vi "robo_preso.vi"(8 "Robot in":T1, 10 "IA State":T6={"our_robots"=[], "enemy_robots"=[], "balls"=[], "geometry"={"field_length"=0, "field_width"=0, "goal_width"=0, "goal_depth"=0, "center_circle_radius"=0, "defense_width"=0, "defense_depth"=0, "free_kick_from_defense_dist"=0, "penalty_spot_from_field_line_dist"=0, "penalty_line_from_spot_dist"=0, "half_moon_depth"=0, "half_moon_width"=0}, "IA Judge"={"stage"="", "command"="", "our_goalie_id"=0.0, "enemy_goalie_id"=0.0, "command enum"=enum."Halt", "Time"=enum."Azul"}, "Received Timestamp"=timestamp(0 s since 1904-01-01), "Events"={"Touch"=FALSE, "id touch"=0.0, "Ball out of \nVision"=FALSE, "Ball inside \nGoalie area"=FALSE, "Robot not responding"=FALSE, "Robots responding status"=[1.0, 1.0, 1.0, 1.0, 1.0, 1.0], "Enemy Ball \nPossession"=FALSE, "Id ini Possession"=0.0, "Ball Possesion"=FALSE, "Id Possesion"=0.0, "Ball at\nour goal side"=FALSE, "Ball at\ntouchline"=FALSE, "Ball at\nenemy goal side"=FALSE}}, 11 "balls":T7[](array[typedef])) -> (1 "result":bool, 3 "Robot out":T1)   [LabVIEW 2018]
uses:
  Core/AI Ball.ctl
  Core/AI Robot.ctl
  Functions Enum.ctl
  AttackerStates.ctl
  Path Planning/RRT/PathDests.ctl
  Path Planning/RRT/PathDest.ctl
  Core/AI Input.ctl
  Core/Field Size.ctl
  Core/AI Judge.ctl
  Command Enum.ctl
  Util/Events/Events.ctl
  <vilib>/Analysis/_algsub.llb/Real Vector Norm.vi
  <vilib>/Analysis/NI_AALPro.lvlib
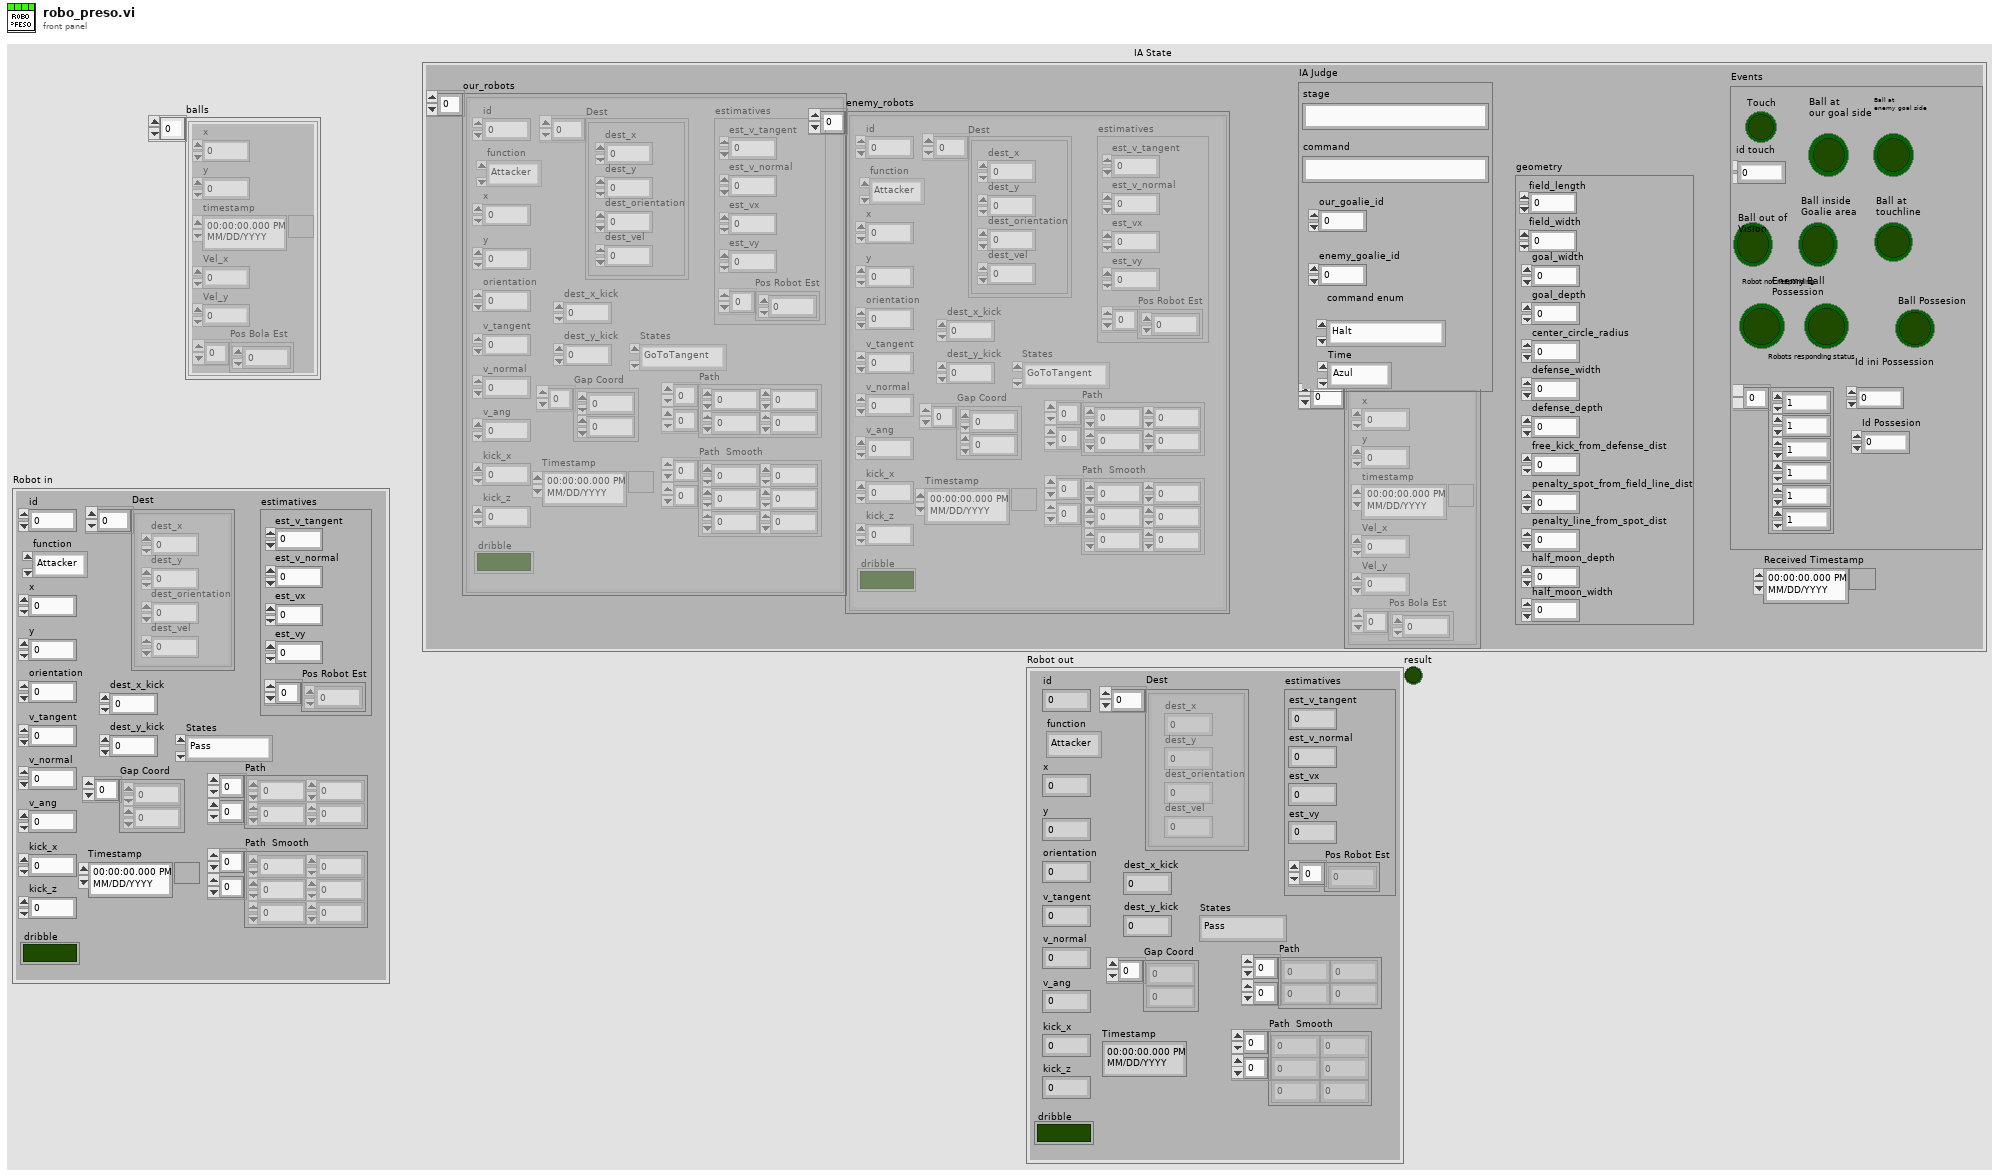
[diagram p1: front panel]
types:
  T1 = typedef "AI Robot.ctl" = cluster{"id":u32, "function":T2, "x":dbl, "y":dbl, "orientation":dbl, "v_tangent":dbl, "v_normal":dbl, "v_ang":dbl, "kick_x":dbl, "kick_z":dbl, "dribble":bool, "Timestamp":timestamp, "estimatives":cluster{"est_v_tangent":dbl, "est_v_normal":dbl, "est_vx":dbl, "est_vy":dbl, "Pos Robot Est":dbl[]}, "dest_x_kick":dbl, "dest_y_kick":dbl, "Gap Coord":dbl[], "States":T3, "Path ":dbl[][], "Path  Smooth":dbl[][], "Dest":T4}
  T2 = typedef "Functions Enum.ctl" = enum16{"Attacker", "Goalie", "Defender", "Striker", "Goto 0", "Dummy", "Kicker", "ZigZag"}
  T3 = typedef "AttackerStates.ctl" = enum16{"Pass", "GoToTangent", "BallGetting", "GoToKick", "Rotate anti-clockwise", "Rotate Clockwise", ""}
  T4 = typedef "PathDests.ctl" = T5[]
  T5 = typedef "PathDest.ctl" = cluster{"dest_x":dbl, "dest_y":dbl, "dest_orientation":dbl, "dest_vel":dbl}
  T6 = typedef "AI Input.ctl" = cluster{"our_robots":T1[], "enemy_robots":T1[], "balls":T7[], "geometry":T8, "IA Judge":T9, "Received Timestamp":timestamp, "Events":T11}
  T7 = typedef "AI Ball.ctl" = cluster{"x":dbl, "y":dbl, "timestamp":timestamp, "Vel_x":dbl, "Vel_y":dbl, "Pos Bola Est":dbl[]}
  T8 = typedef "Field Size.ctl" = cluster{"field_length":u32, "field_width":u32, "goal_width":u32, "goal_depth":u32, "center_circle_radius":u32, "defense_width":u32, "defense_depth":u32, "free_kick_from_defense_dist":u32, "penalty_spot_from_field_line_dist":u32, "penalty_line_from_spot_dist":u32, "half_moon_depth":u32, "half_moon_width":u32}
  T9 = typedef "AI Judge.ctl" = cluster{"stage":string, "command":string, "our_goalie_id":dbl, "enemy_goalie_id":dbl, "command enum":T10, "Time":enum16{"Azul", "Amarelo"}}
  T10 = typedef "Command Enum.ctl" = enum16{"Halt", "Stop", "Force Start", "PKA Normal Start", "Prepare Kickoff Ally", "PKE Normal Start", "Prepare Kickoff Enemy", "Prepare Penalty Ally", "PPA Normal Start", "Prepare Penalty Enemy", "PPE Normal Start", "Ball Placement Enemy Up", "Ball Placement Enemy Down", "Ball Placement Ally Up", "Ball Placement Ally Mid", "Ball Placement Ally Down", "Indirect Free Enemy", "Indirect Free Ally", "Timeout Enemy", "Timeout Ally", "Goal Enemy", "Goal Ally", "Normal Half Time", "Extra Time Break", "Extra Half Time", "None", "Post Game"}
  T11 = typedef "Events.ctl" = cluster{"Touch":bool, "id touch":dbl, "Ball out of \nVision":bool, "Ball inside \nGoalie area":bool, "Robot not responding":bool, "Robots responding status":dbl[], "Enemy Ball \nPossession":bool, "Id ini Possession":dbl, "Ball Possesion":bool, "Id Possesion":dbl, "Ball at\nour goal side":bool, "Ball at\ntouchline":bool, "Ball at\nenemy goal side":bool}
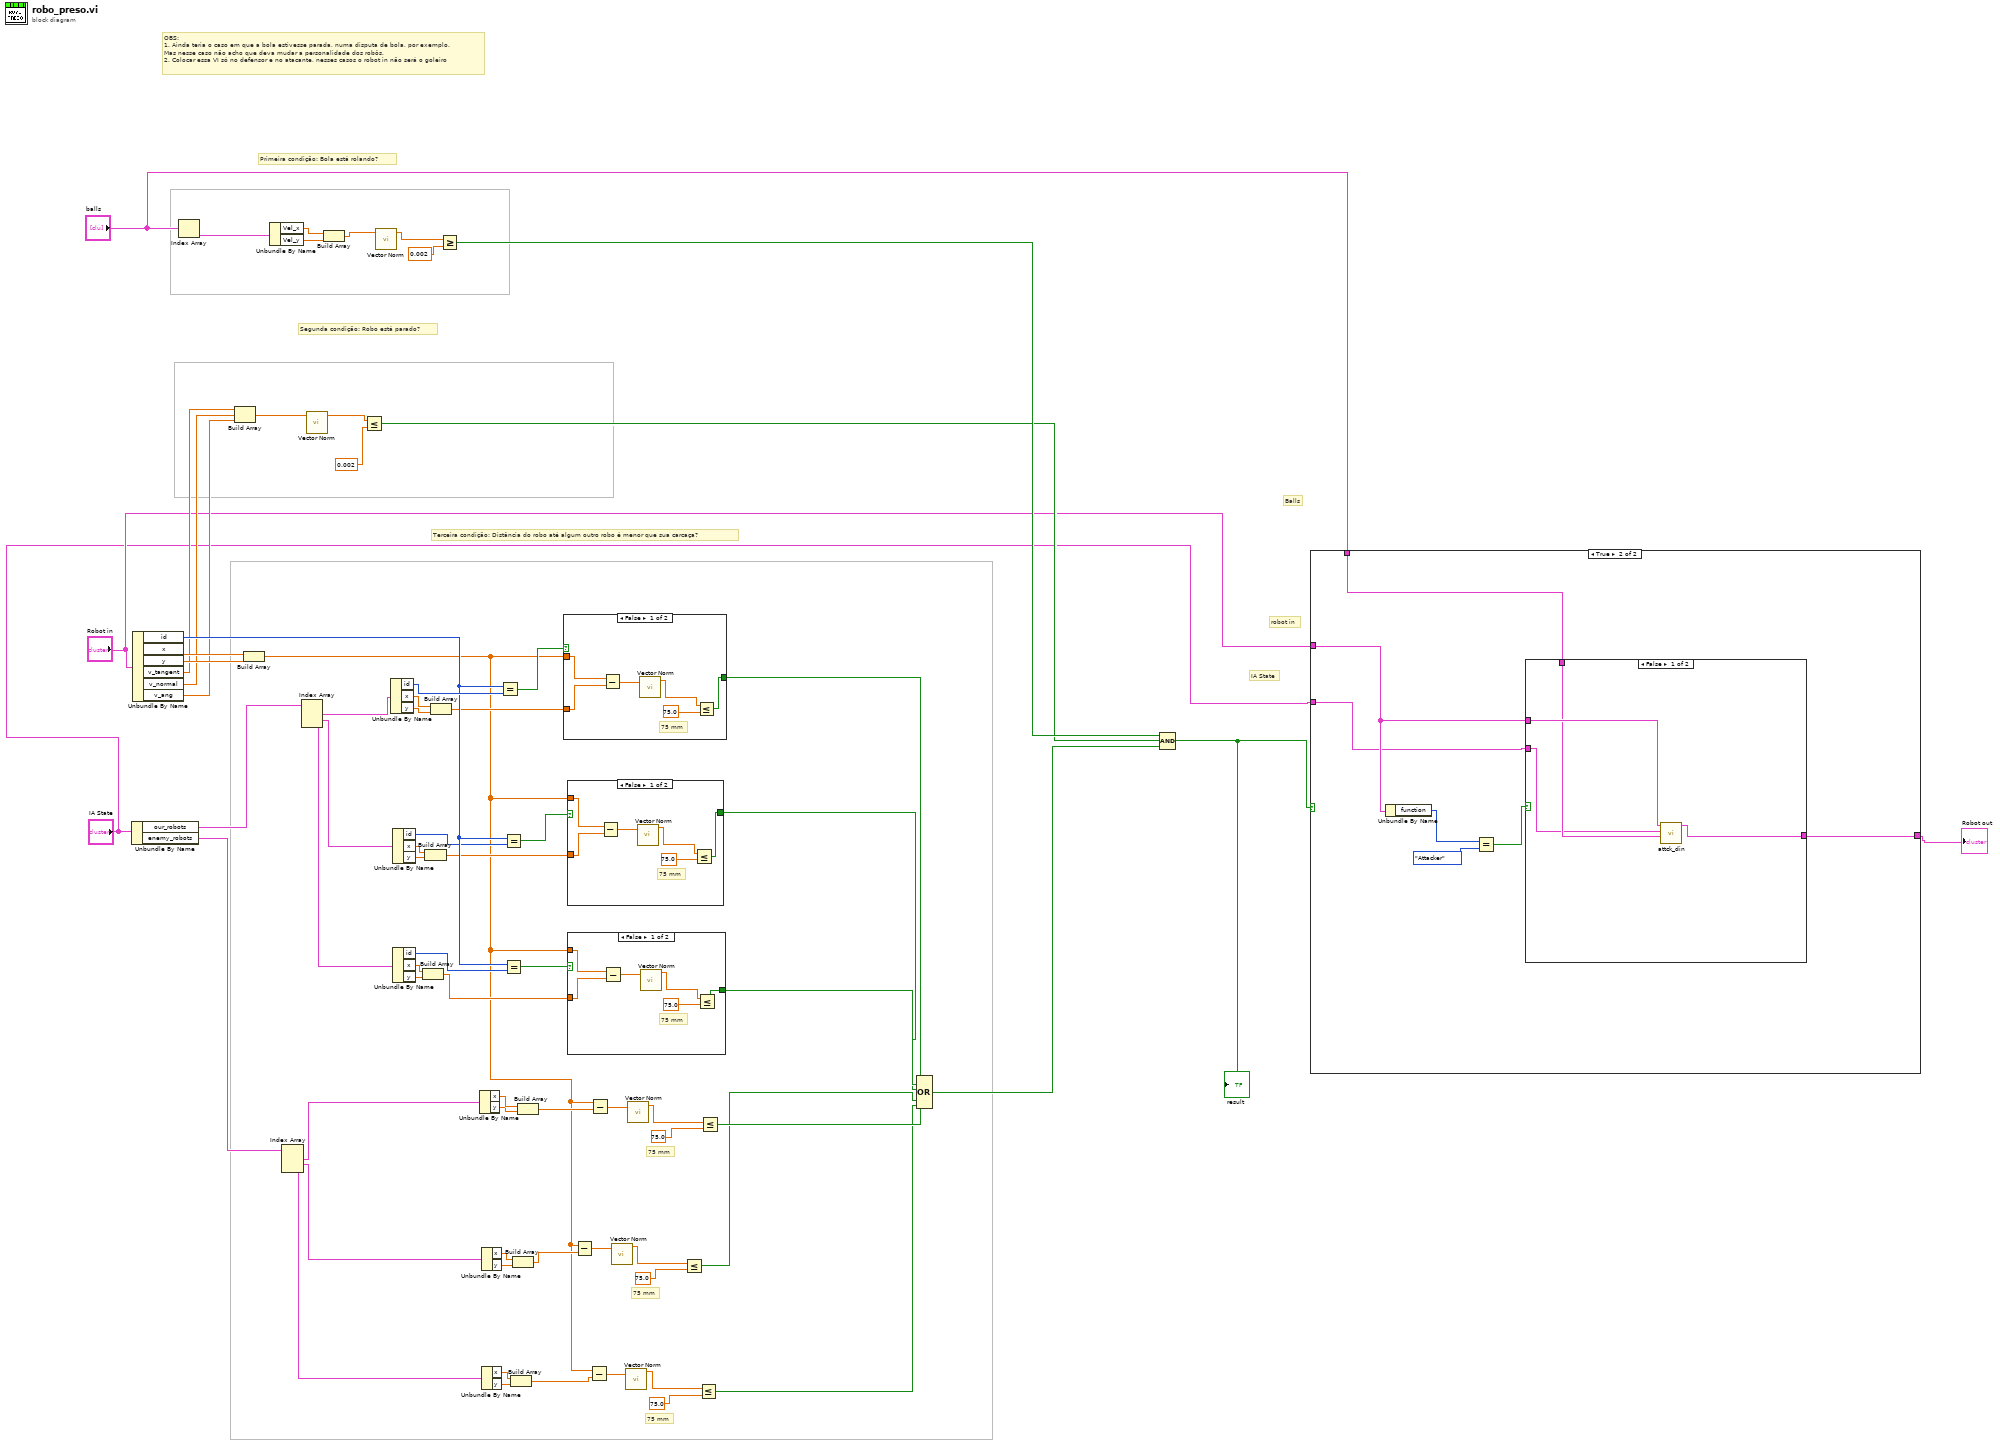
[diagram p0: block diagram]
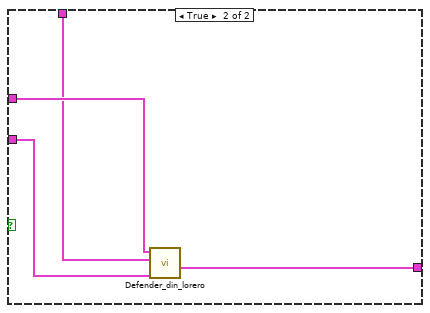
[diagram p3: hidden frame]
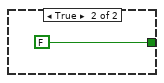
[diagram p4: hidden frame]
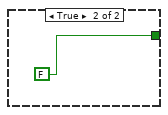
[diagram p5: hidden frame]
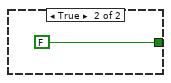
[diagram p6: hidden frame]
diagram:
  # "IA State"
  # "Balls"
  # "robot in"
  # "OBS:\n1. Ainda teria o caso em que a bola estivesse parada, numa disputa de bola, por exemplo.\nMas nesse caso não acho que deva mudar a personalidade dos robôs.\n2. Colocar essa VI só no defensor e no atacante, nesses casos o robot in não será o goleiro"
  # "Segunda condição: Robo está parado?"
  # "75 mm"
  # "75 mm"
  # "75 mm"
  # "Terceira condição: Distância do robo até algum outro robo é menor que sua carcaça?"
  # "Primeira condição: Bola está rolando?"
  n1 = Unbundle By Name("IA State") -> ("our_robots"=w5:T1[], "enemy_robots"=w33:T1[])
  n2 = Unbundle By Name("Robot in") -> ("id"=w60:u32, "x"=w54:dbl, "y"=w53:dbl, "v_tangent"=w14:dbl, "v_normal"=w13:dbl, "v_ang"=w12:dbl)
  n3 = Index Array(array="balls") -> (element=w71:T7)  [unwired: 1 in]
  n4 = Build Array(w14, w13, w12) -> (w11:dbl[])
  n5 = Build Array(w54, w53) -> (w19:dbl[])
  n6 = Unbundle By Name(w71) -> ("Vel_x"=w70:dbl, "Vel_y"=w69:dbl)
  n7 = Index Array(array=w33) -> (element #1=w34:T1, element #2=w32:T1, element #3=w31:T1)  [unwired: 3 in]
  n8 = Index Array(array=w5) -> (element #1=w62:T1, element #2=w64:T1, element #3=w63:T1)  [unwired: 3 in]
  n9 = call-poly <vilib>:"Vector Norm.vi"("Input Vector"=w11) -> ("norm"=w9:dbl)  [unwired: 9 in, 1 out]
  n10 = Build Array(w70, w69) -> (w68:dbl[])
  n11 = Less Or Equal?(x=w9, y=0.002) -> (x <= y?=w7:bool)
  n12 = call-poly <vilib>:"Vector Norm.vi"("Input Vector"=w68) -> ("norm"=w67:dbl)  [unwired: 9 in, 1 out]
  n13 = Unbundle By Name(w62) -> ("id"=w61:u32, "x"=w52:dbl, "y"=w51:dbl)
  n14 = Unbundle By Name(w64) -> ("id"=w59:u32, "x"=w50:dbl, "y"=w49:dbl)
  n15 = Unbundle By Name(w63) -> ("id"=w58:u32, "x"=w48:dbl, "y"=w47:dbl)
  n16 = Build Array(w48, w47) -> (w44:dbl[])
  n17 = Build Array(w50, w49) -> (w45:dbl[])
  n18 = Build Array(w52, w51) -> (w46:dbl[])
  n19 = Greater Or Equal?(x=w67, y=0.002) -> (x >= y?=w65:bool)
  n20 = Unbundle By Name(w34) -> ("x"=w40:dbl, "y"=w39:dbl)
  n21 = Unbundle By Name(w32) -> ("x"=w38:dbl, "y"=w37:dbl)
  n22 = Unbundle By Name(w31) -> ("x"=w36:dbl, "y"=w35:dbl)
  n23 = Equal?(x=w60, y=w61) -> (x = y?=w57:bool)
  n24 = Equal?(x=w60, y=w59) -> (x = y?=w56:bool)
  n25 = Equal?(x=w60, y=w58) -> (x = y?=w55:bool)
  n26 = Build Array(w36, w35) -> (w18:dbl[])
  n27 = Build Array(w38, w37) -> (w20:dbl[])
  n28 = Build Array(w40, w39) -> (w29:dbl[])
  n29 = case shown="False" w57 {
    tunnel: w19 -> [w77 _]
    tunnel: w46 -> [w76 _]
    tunnel: [w72 FALSE] -> w43
    frame False {
      # "75 mm"
      n30 = Subtract(x=w77, y=w76) -> (x-y=w75:dbl[])
      n31 = call-poly <vilib>:"Vector Norm.vi"("Input Vector"=w75) -> ("norm"=w74:dbl)  [unwired: 9 in, 1 out]
      n32 = Less Or Equal?(x=w74, y=75.0) -> (x <= y?=w72:bool)
    }
    frame True {
    }
  }
  n33 = case shown="False" w55 {
    tunnel: w19 -> [w81 _]
    tunnel: w44 -> [w80 _]
    tunnel: [w79 FALSE] -> w41
    frame False {
      # "75 mm"
      n34 = Subtract(x=w81, y=w80) -> (x-y=w83:dbl[])
      n35 = call-poly <vilib>:"Vector Norm.vi"("Input Vector"=w83) -> ("norm"=w84:dbl)  [unwired: 9 in, 1 out]
      n36 = Less Or Equal?(x=w84, y=75.0) -> (x <= y?=w79:bool)
    }
    frame True {
    }
  }
  n37 = case shown="False" w56 {
    tunnel: w19 -> [w88 _]
    tunnel: w45 -> [w87 _]
    tunnel: [w86 FALSE] -> w42
    frame False {
      # "75 mm"
      n38 = Subtract(x=w88, y=w87) -> (x-y=w90:dbl[])
      n39 = call-poly <vilib>:"Vector Norm.vi"("Input Vector"=w90) -> ("norm"=w91:dbl)  [unwired: 9 in, 1 out]
      n40 = Less Or Equal?(x=w91, y=75.0) -> (x <= y?=w86:bool)
    }
    frame True {
    }
  }
  n41 = Subtract(x=w19, y=w20) -> (x-y=w26:dbl[])
  n42 = Subtract(x=w19, y=w18) -> (x-y=w23:dbl[])
  n43 = Subtract(x=w19, y=w29) -> (x-y=w30:dbl[])
  n44 = call-poly <vilib>:"Vector Norm.vi"("Input Vector"=w26) -> ("norm"=w25:dbl)  [unwired: 9 in, 1 out]
  n45 = call-poly <vilib>:"Vector Norm.vi"("Input Vector"=w23) -> ("norm"=w22:dbl)  [unwired: 9 in, 1 out]
  n46 = call-poly <vilib>:"Vector Norm.vi"("Input Vector"=w30) -> ("norm"=w28:dbl)  [unwired: 9 in, 1 out]
  n47 = Less Or Equal?(x=w25, y=75.0) -> (x <= y?=w16:bool)
  n48 = Less Or Equal?(x=w22, y=75.0) -> (x <= y?=w15:bool)
  n49 = Less Or Equal?(x=w28, y=75.0) -> (x <= y?=w17:bool)
  n50 = Compound Arithmetic op=OR(w43, w42, w41, w17, w16, w15) -> (w8:bool)
  n51 = Compound Arithmetic op=AND(w65, w7, w8) -> (w6:bool)
  "result" <- w6
  n52 = case shown="True" w6 {
    tunnel: "Robot in" -> [w93 w97]
    tunnel: "balls" -> [_ w96]
    tunnel: "IA State" -> [_ w95]
    tunnel: [w93 w94] -> w1
    frame False {
    }
    frame True {
      n53 = Unbundle By Name(w97) -> ("function"=w100:T2)
      n54 = Equal?(x=w100, y=Functions_Enum."Attacker") -> (x = y?=w98:bool)
      n55 = case shown="False" w98 {
        tunnel: w97 -> [w104 w108]
        tunnel: w96 -> [w103 w107]
        tunnel: w95 -> [w102 w106]
        tunnel: [w101 w105] -> w94
        frame False {
          n56 = call "attck_din.vi"("balls"=w103, "IA State"=w102, "Robot in"=w104) -> ("Robot out"=w101:T1)  [unwired: 8 in]
        }
        frame True {
          n57 = call "Defender_din_lorero.vi"("IA State"=w106, "balls"=w107, "Robot in"=w108) -> ("Robot out"=w105:T1)  [unwired: 8 in]
        }
      }
    }
  }
  "Robot out" <- w1
